vi "任意角度矩形框绘制_子VI.vi"(10 "任意角度矩形框各顶点坐标值":T2, 11 "Image":T1) -> (3 "Image Out":T1)   [LabVIEW 2018]
uses:
  <vilib>/vision/Image Controls.llb/IMAQ Image.ctl
  <vilib>/vision/NI_Vision_Development_Module.lvlib
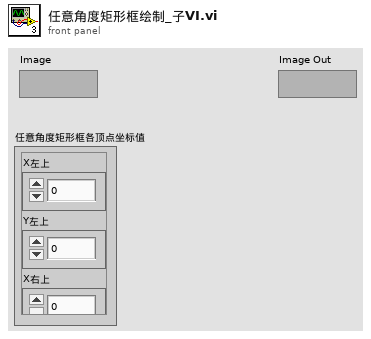
[diagram p1: front panel]
types:
  T1 = typedef "IMAQ Image.ctl" = refnum<image>
  T2 = cluster{"X左上":i32, "Y左上":i32, "X右上":i32, "Y右上":i32, "X左下":i32, "Y左下":i32, "X右下":i32, "Y右下":i32}
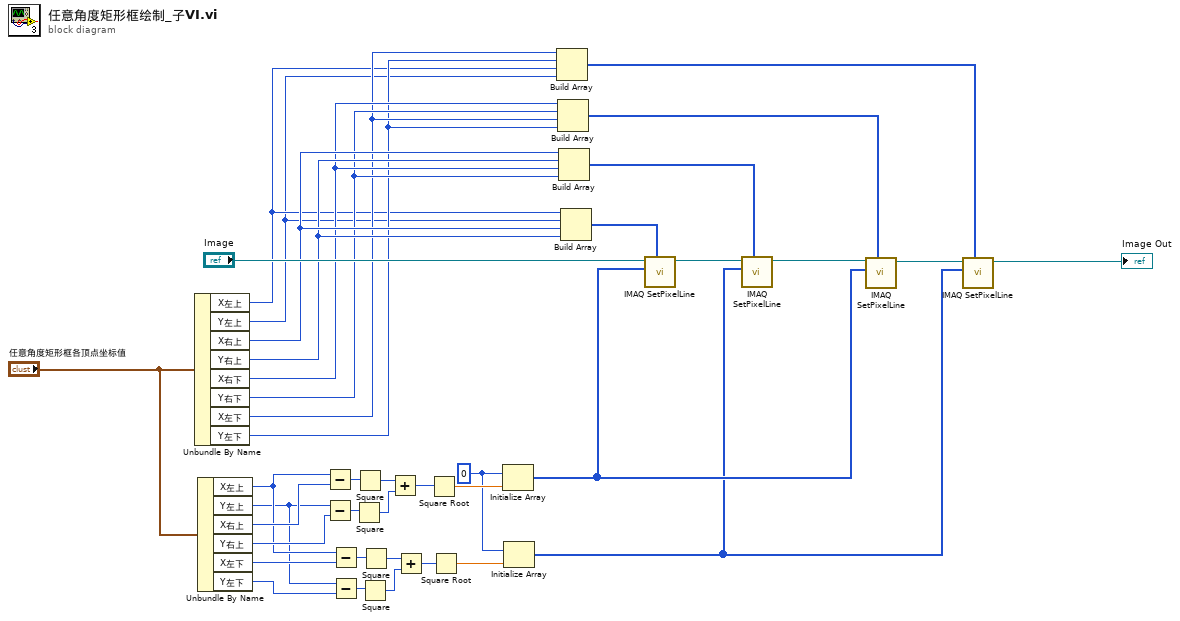
[diagram p0: block diagram]
diagram:
  w19 = u8 0 ("元素")
  n1 = Unbundle By Name("任意角度矩形框各顶点坐标值") -> ("X左上"=w2:i32, "Y左上"=w1:i32, "X右上"=w8:i32, "Y右上"=w7:i32, "X右下"=w6:i32, "Y右下"=w5:i32, "X左下"=w4:i32, "Y左下"=w3:i32)
  n2 = Unbundle By Name("任意角度矩形框各顶点坐标值") -> ("X左上"=w28:i32, "Y左上"=w26:i32, "X右上"=w38:i32, "Y右上"=w35:i32, "X左下"=w27:i32, "Y左下"=w25:i32)
  n3 = Subtract(x=w28, y=w38) -> (x-y=w37:i32)
  n4 = Subtract(x=w26, y=w35) -> (x-y=w34:i32)
  n5 = Subtract(x=w28, y=w27) -> (x-y=w29:i32)
  n6 = Subtract(x=w26, y=w25) -> (x-y=w31:i32)
  n7 = Square(x=w34) -> (x^2=w33:i32)
  n8 = Square(x=w37) -> (x^2=w36:i32)
  n9 = Square(x=w31) -> (x^2=w32:i32)
  n10 = Square(x=w29) -> (x^2=w30:i32)
  n11 = Add(x=w36, y=w33) -> (x+y=w23:i32)
  n12 = Add(x=w30, y=w32) -> (x+y=w22:i32)
  n13 = Square Root(x=w23) -> (sqrt(x)=w21:dbl)
  n14 = Square Root(x=w22) -> (sqrt(x)=w20:dbl)
  n15 = Initialize Array(w19, w21) -> (w14:u8[])
  n16 = Initialize Array(w19, w20) -> (w13:u8[])
  n17 = Build Array(w4, w3, w2, w1) -> (w9:i32[])
  n18 = Build Array(w6, w5, w4, w3) -> (w10:i32[])
  n19 = Build Array(w8, w7, w6, w5) -> (w11:i32[])
  n20 = Build Array(w2, w1, w8, w7) -> (w12:i32[])
  n21 = call "IMAQ SetPixelLine"("Line Coordinates"=w12, "Pixels Line (U8)"=w14, "Image"="Image") -> ("Image Out"=w18:T1)  [unwired: 7 in, 1 out]
  n22 = call "IMAQ SetPixelLine"("Line Coordinates"=w11, "Pixels Line (U8)"=w13, "Image"=w18) -> ("Image Out"=w17:T1)  [unwired: 7 in, 1 out]
  n23 = call "IMAQ SetPixelLine"("Line Coordinates"=w10, "Pixels Line (U8)"=w14, "Image"=w17) -> ("Image Out"=w16:T1)  [unwired: 7 in, 1 out]
  n24 = call "IMAQ SetPixelLine"("Line Coordinates"=w9, "Pixels Line (U8)"=w13, "Image"=w16) -> ("Image Out"=→"Image Out":T1)  [unwired: 7 in, 1 out]
